vi "OptællingsArray.vi"(11 "Numeric":i32) -> (3 "Array":i32[](array[numeric]))   [LabVIEW 2022 SP3]
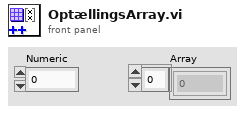
[diagram p1: front panel]
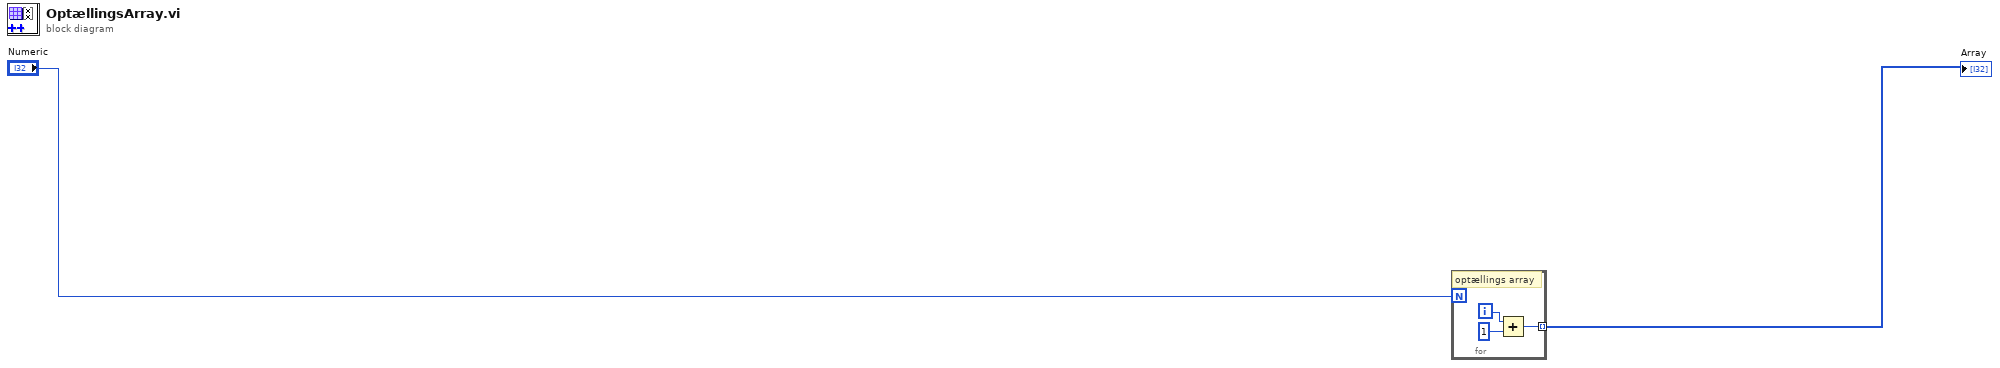
[diagram p0: block diagram]
diagram:
  n1 = for {
    N: "Numeric" -> [_]
    tunnel: [w3] -> w2 mode=indexing
    i -> [w5]
    # "optællings array"
    n2 = Add(x=w5, y=1) -> (x+y=w3:i32)
  }
  "Array" <- w2
